vi "Ex8 Morphological Operations.vi"() -> ()   [LabVIEW 2020]
panel:
  in  "Square/Hexa (Square)":bool
  in  "Structuring Element":i32[][](array[numeric])=[[0, 0, 0, 1, 1, 1, 1, 1, 0, 0, 0], [0, 0, 1, 1, 1, 1, 1, 1, 1, 0, 0], [0, 1, 1, 1, 1, 1, 1, 1, 1, 1, 0], [1, 1, 1, 1, 1, 1, 1, 1, 1, 1, 1], [1, 1, 1, 1, 1, 1, 1, 1, 1, 1, 1], [1, 1, 1, 1, 1, 1, 1, 1, 1, 1, 1], [1, 1, 1, 1, 1, 1, 1, 1, 1, 1, 1], [1, 1, 1, 1, 1, 1, 1, 1, 1, 1, 1], [0, 1, 1, 1, 1, 1, 1, 1, 1, 1, 0], [0, 0, 1, 1, 1, 1, 1, 1, 1, 0, 0], [0, 0, 0, 1, 1, 1, 1, 1, 0, 0, 0]]
  in  "Number of iterations":i32=1
  in  "Operation":T1(ring)=enum."Dilate"
  out "error out":errorcluster
  out "Image":T2(plugin-control)
  in  "File Path":path
  out "Processed Image":T2(plugin-control)
  # "EX.8 MORPHOLOGICAL OPERATIONS"
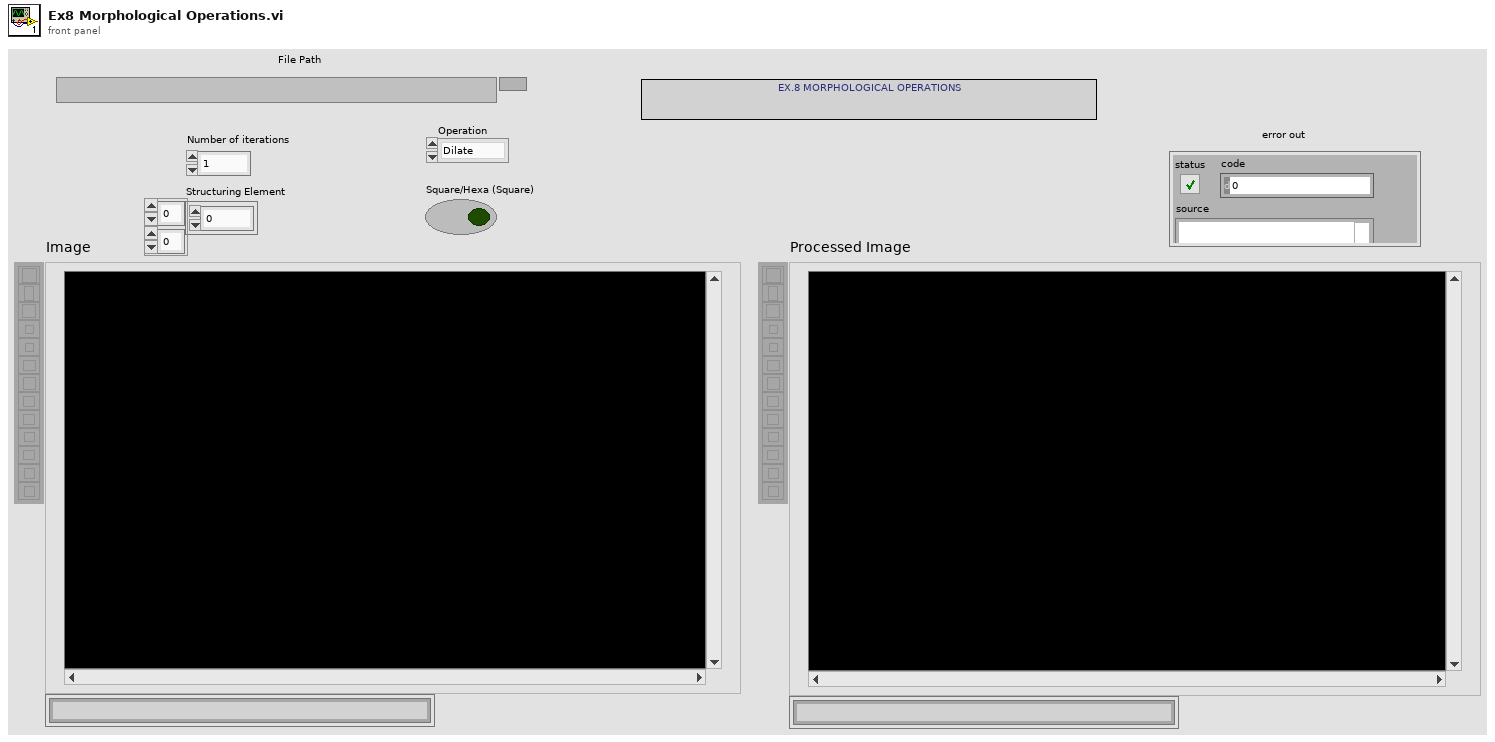
[diagram p1: front panel]
types:
  T1 = enum32{"AutoM", "Close", "Dilate", "Erode", "Gradient", "Gradient out", "Gradient in", "Hit miss", "Open", "PClose", "POpen", "Thick", "Thin"}
  T2 = typedef "IMAQ Image.ctl" = refnum<image>
  T3 = typedef "Image Type" = u32
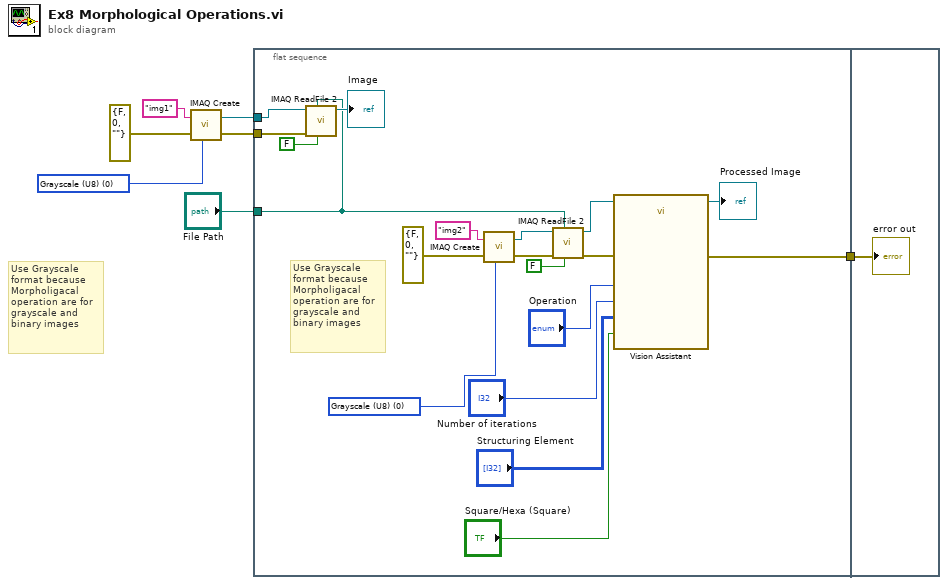
[diagram p0: block diagram]
diagram:
  w1 = T3 0 items=["Grayscale (U8)", "Grayscale (I16)", "Grayscale (SGL)", "Complex (CSG)", "RGB (U32)", "HSL (U32)", "RGB (U64)", "Grayscale (U16)"] ("Image Type")
  # "Use Grayscale format because Morpholigacal operation are for grayscale and binary images"
  n1 = call "IMAQ Create"("Image Name"="img1", "Image Type"=w1, "error in (no error)"=errorcluster {"status"=FALSE, "code"=0, "source"=""}) -> ("New Image"=w2:T2, "error out"=w3:errorcluster)  [unwired: 2 in]
  n2 = flat-sequence {
    tunnel: "File Path" -> [w16]
    tunnel: w3 -> [w25]
    tunnel: w2 -> [w24]
    tunnel: [w12] -> w7
    tunnel: w7 -> [w27]
    frame #0 {
      w20 = T3 0 items=["Grayscale (U8)", "Grayscale (I16)", "Grayscale (SGL)", "Complex (CSG)", "RGB (U32)", "HSL (U32)", "RGB (U64)", "Grayscale (U16)"] ("Image Type")
      # "Use Grayscale format because Morpholigacal operation are for grayscale and binary images"
      n3 = call "IMAQ ReadFile 2"("Use File Path Image Type"=FALSE, "File Path"=w16, "error in (no error)"=w25, "Image"=w24) -> ("Image Out"=→"Image":T2)  [unwired: 3 in, 4 out]
      n4 = call "IMAQ Create"("Image Name"="img2", "Image Type"=w20, "error in (no error)"=errorcluster {"status"=FALSE, "code"=0, "source"=""}) -> ("New Image"=w19:T2, "error out"=w18:errorcluster)  [unwired: 2 in]
      n5 = call "IMAQ ReadFile 2"("Use File Path Image Type"=FALSE, "File Path"=w16, "error in (no error)"=w18, "Image"=w19) -> ("error out"=w14:errorcluster, "Image Out"=w15:T2)  [unwired: 3 in, 3 out]
      n6 = call "Vision Assistant"("Image In"=w15, "Operation (Basic Morphology 1)"="Operation", "Number of iterations (1) (Basic Morphology 1)"="Number of iterations", "Structuring Element (Basic Morphology 1)"="Structuring Element", "Square/Hexa (Square) (Basic Morphology 1)"="Square/Hexa (Square)", "error in"=w14) -> ("Image Out"=→"Processed Image":T2, "error out"=w12:errorcluster)  [unwired: 20 in]
    }
    frame #1 {
      "error out" <- w27
    }
  }
